vi "Get Reply Data.vi"(8 "error in (no error)":errorcluster, 9 "Data Msg in":refnum<class "Data Msg.lvclass">, 10 "Actor in":refnum<class "Actor.lvclass">, 11 "ReplayData Message":refnum<class "Get Parameter Msg.lvclass">) -> (0 "error out":errorcluster, 1 "Data Msg out":refnum<class "Data Msg.lvclass">, 2 "Actor out":refnum<class "Actor.lvclass">, 3 "ReplayData Message out":refnum<class "Get Parameter Msg.lvclass">, 4 "error?":bool)   [LabVIEW 2014, in "Get Parameter Msg.lvclass"]
doc: "(<B>Filename</B>: Actor Framework.lvlib:Message.lvclass:Do.vi)\n\nDefines what a message does when it is received by an actor. Generally, a message instructs an actor to invoke one of its methods. By default, this method does nothing. A child class must override it to define behavior. Create a child class by using the Actor Framework Message Maker dialog box."
uses:
  Get Parameter Msg.lvclass
  <vilib>/ActorFramework/Actor/Actor.lvclass
  Model/Data Msg/Data Msg.lvclass
  ParameterDevice.lvclass
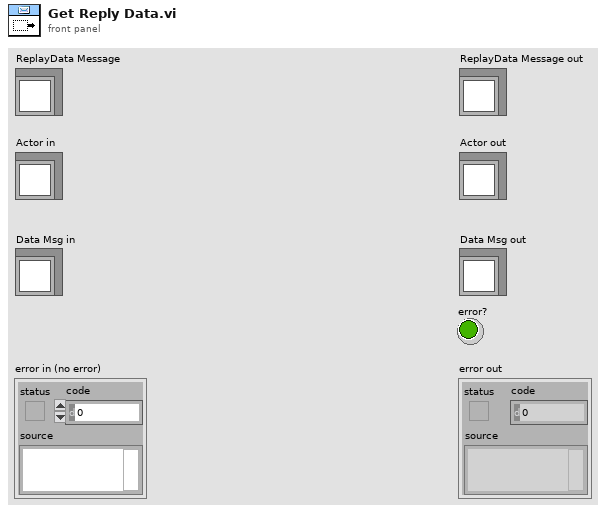
[diagram p1: front panel]
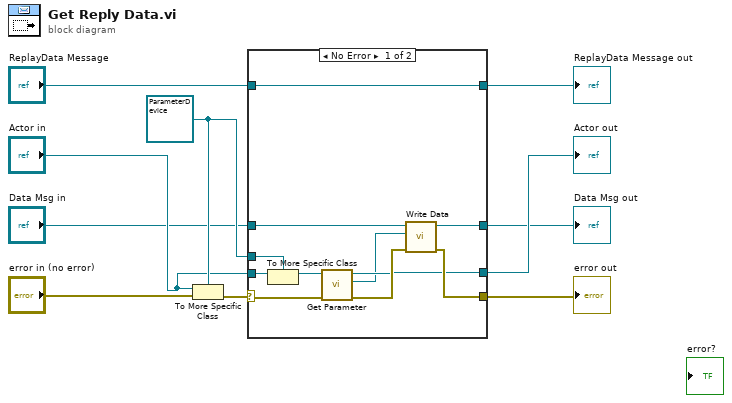
[diagram p0: block diagram]
diagram:
  w9 = refnum<class "ParameterDevice.lvclass"> refnum ("Actor in")
  n1 = To More Specific Class(target class=w9, reference="Actor in", error in="error in (no error)") -> (error out=w10:errorcluster)  [unwired: 1 out]
  n2 = case shown="No Error" w10 {
    selector: w10 -> [w11 w25]
    tunnel: [w17 w25] -> w8
    tunnel: [w16 w24] -> w3
    tunnel: "Actor in" -> [w21 w24]
    tunnel: w9 -> [w20 _]
    tunnel: "ReplayData Message" -> [w15 w22]
    tunnel: "Data Msg in" -> [w19 w23]
    tunnel: [w15 w22] -> w2
    tunnel: [w14 w23] -> w1
    frame No Error {
      n3 = To More Specific Class(target class=w20, reference=w21) -> (specific class reference=w12:refnum<class "ParameterDevice.lvclass">)  [unwired: 1 in, 1 out]
      n4 = call-dynamic "Get Parameter.vi"("error in (no error)"=w11, "ParameterDevice in"=w12) -> ("error out"=w18:errorcluster, "Parameter"=w13:refnum<class "AbstractData.lvclass">, "ParameterDevice out"=w16:refnum<class "ParameterDevice.lvclass">)  [unwired: 7 in]
      n5 = call-dynamic "Write Data.vi"("error in (no error)"=w18, "AbstractData.lvclass"=w13, "Data Msg in"=w19) -> ("error out"=w17:errorcluster, "Data Msg out"=w14:refnum<class "Data Msg.lvclass">)  [unwired: 7 in]
    }
    frame Error {
      # "If type check fails, pass the original object out again."
    }
  }
  "error out" <- w8
  "Actor out" <- w3
  "ReplayData Message out" <- w2
  "Data Msg out" <- w1
